vi "Get TextDocument Refnum.vi"(8 "error in (no error)":errorcluster, 11 "ooCalc in":refnum<class "ooCalc.lvclass">) -> (0 "error out":errorcluster, 2 "SpreadsheetDocument":refnum<k24>, 3 "ooCalc out":refnum<class "ooCalc.lvclass">)   [LabVIEW 2009, in "ooCalc.lvclass"]
uses:
  ooCalc.lvclass
  C:/Projets/LAVAG/OpenOfficeRGT/AODL/DLLs/AODL.dll
  ooCalc.lvclass/ooCalc.ctl
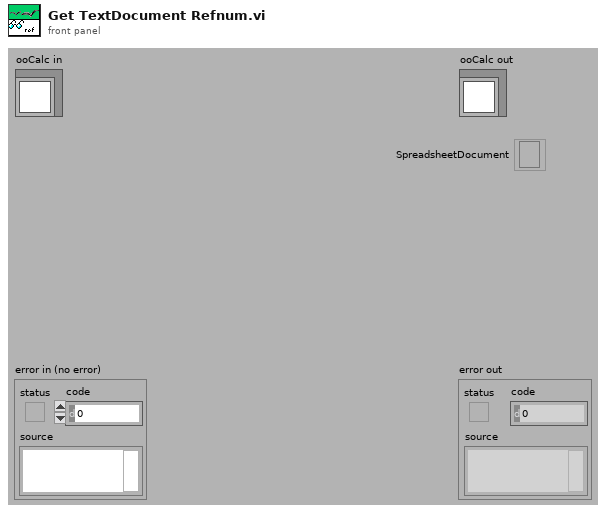
[diagram p1: front panel]
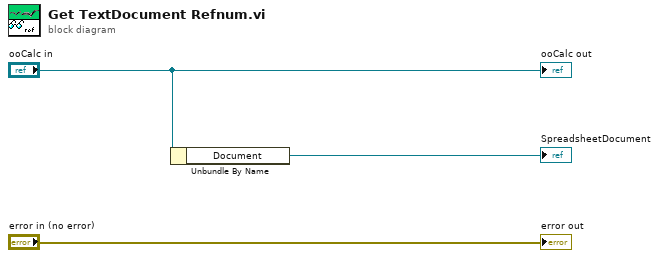
[diagram p0: block diagram]
diagram:
  n1 = Unbundle By Name("ooCalc in") -> ("Document"=→"SpreadsheetDocument":refnum<k24>)
  "error out" <- "error in (no error)"
  "ooCalc out" <- "ooCalc in"
